vi "Loop Async.vi"(10 "ExecAnchor":refnum<class "ExecAnchor.lvclass">, 11 "GroupLoggingControl in":refnum<class "GroupLoggingControl.lvclass">) -> ()   [LabVIEW 2020, in "VolatusGUIElements.lvlib" / "GroupLoggingControl.lvclass"]
uses:
  GroupLoggingControl.lvclass
  GroupLoggingControl.lvclass/GroupLoggingControl.ctl
  lv-exec-anchor/ExecAnchor/ExecAnchor.lvclass
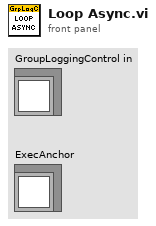
[diagram p1: front panel]
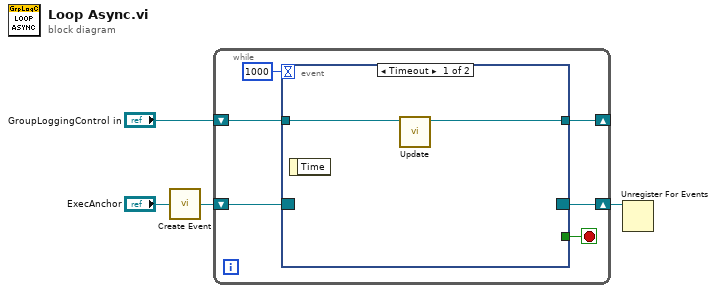
[diagram p0: block diagram]
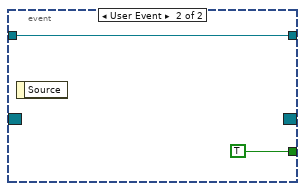
[diagram p2: hidden frame]
diagram:
  n1 = call "Create Event.vi"("ExecAnchor in"="ExecAnchor") -> ("Event Reg"=w3:refnum<event-registration>)  [unwired: 3 in, 1 out]
  n2 = while {
    shift-right: [w8] -> w1
    shift-left: w3 -> [w9]
    shift-right: [w6] -> _
    shift-left: "GroupLoggingControl in" -> [w5]
    stop <- w7 stop-if-true
    n3 = event shown="[0] Timeout" {
      selector: w9 -> [_ _]
      dyn-events: [_ _] -> w8
      timeout: 1000 -> [_ _]
      tunnel: [_ TRUE] -> w7
      tunnel: [w11 w13] -> w6
      tunnel: w5 -> [w12 w13]
      event Timeout {
        n4 = event-data() -> ()  [unwired: 1 in, 1 out]
        n5 = call "Update.vi"("GroupLoggingControl in"=w12) -> ("GroupLoggingControl out"=w11:refnum<class "GroupLoggingControl.lvclass">)  [unwired: 9 in, 1 out]
      }
      event User Event {
        n6 = event-data() -> ()  [unwired: 1 in, 1 out]
      }
    }
  }
  n7 = Unregister For Events(event registration refnum=w1) -> ()  [unwired: 1 in, 1 out]
